vi "Fcurve_Create.vi"(0 "reference in":refnum<class "Fcurve.lvclass">, 1 "object name":string="Fcurve", 2 "Group metadata":T1, 5 "error in (no error)":errorcluster) -> (14 "reference out":refnum<class "Fcurve.lvclass">, 19 "error out":errorcluster)   [LabVIEW 2019, in "Fcurve.lvclass"]
doc: "Constructor."
uses:
  Fcurve.lvclass
  C:/Program Files (x86)/National Instruments/LabVIEW 2019/vi.lib/addons/_AddQ/G#Object/G#Object.lvclass
  TDMS_DataHandler_class/Fcurve Meta data.ctl
  <vilib>/addons/_AddQ/G#Object/utils/G#Object_CreateMethod.ctl
  <vilib>/addons/_AddQ/G#Object/G#Object.lvclass
  metadata_class/metadata.lvclass
  TDMS_DataHandler_class/TDMS_DataHandler.lvclass
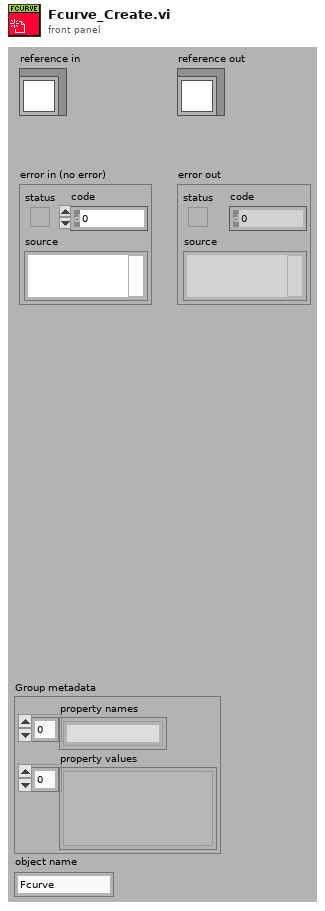
[diagram p1: front panel]
types:
  T1 = typedef "TDMS_DataHandler.lvclass/Fcurve Meta data.ctl" = cluster{"property names":string[], "property values":variant[]}
  T2 = typedef "G#Object.lvclass/G#Object_CreateMethod.ctl" = enum16{"Create", "Create or look up existing", "Look up existing"}
  T3 = typedef "Fcurve.lvclass/ObjectAttributesRef.ctl" = refnum<data-value>
  T4 = typedef "Fcurve.lvclass/ObjectAttributes.ctl" = cluster{"MyAttribute":dbl, "Fcurve Metadata":T5, "Contact Spread of dev":dbl, "Tau Delay (ms)":dbl, "Points of contact":dbl, "Def_wfm":cluster{"Max":dbl, "Min":dbl}, "Zpos_wfm":cluster{"Max":dbl, "Min":dbl}, "Contact stat?":bool, "Real AI dt (s)":dbl, "Decimation":cluster{"App":cluster{"Dec":i32, "apply":bool}, "Con":cluster{"Dec":i32, "apply":bool}, "Ret":cluster{"Dec":i32, "apply":bool}}, "Segment def[0]":dbl, "Segment Zpos[0]":dbl, "Raw Datum":waveform(dbl)[], "Group metadata":T1, "M_data obj":refnum<class "metadata.lvclass">, "Channel name(s)":string[], "Segment fcurve data":cluster{"X":dbl[], "Y":dbl[]}[], "Segment duration":cluster{"Start":i32, "Duration":i32}[], "Segment info":T6[], "Segment durations (S)":dbl[], "Segments Maxmin":T8[]}
  T5 = typedef "Fcurve.lvclass/Metadata.ctl" = cluster{"dt (us)":dbl, "Dec Factor":dbl, "Z piezo Sensitivity (nm/V)":dbl, "K (N/m)":dbl, "Sp (V)":dbl, "Contact (ms)":dbl, "Zpos contact":dbl, "Vel_app (nm/s)":dbl, "Vel_ret (nm/s)":dbl, "deltaV (nm)":dbl, "Def_V0 (v)":dbl, "Piezo gain":dbl, "invOLS (nm/V)":dbl}
  T6 = typedef "Fcurve.lvclass/Fcurve segments --cluster.ctl" = cluster{"type":T7, "nb points":i32, "dec factor":u32, "sampling rate (S/s)":u32}
  T7 = typedef "metadata.lvclass/Segment type--combobox.ctl" = string
  T8 = typedef "Fcurve.lvclass/Segment MaxMin --cluster.ctl" = cluster{"Def":cluster{"max value":dbl, "min value":dbl}, "Zpos":cluster{"max value":dbl, "min value":dbl}}
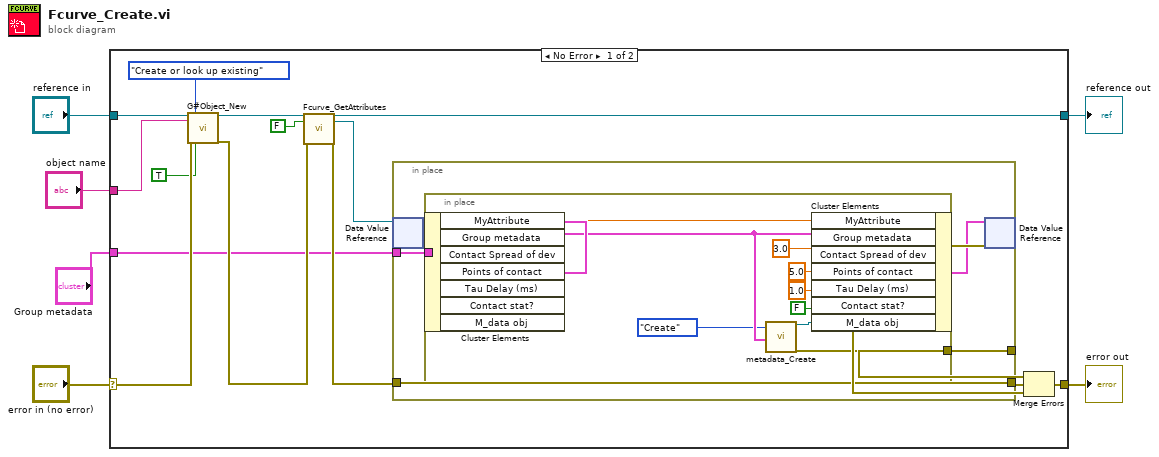
[diagram p0: block diagram]
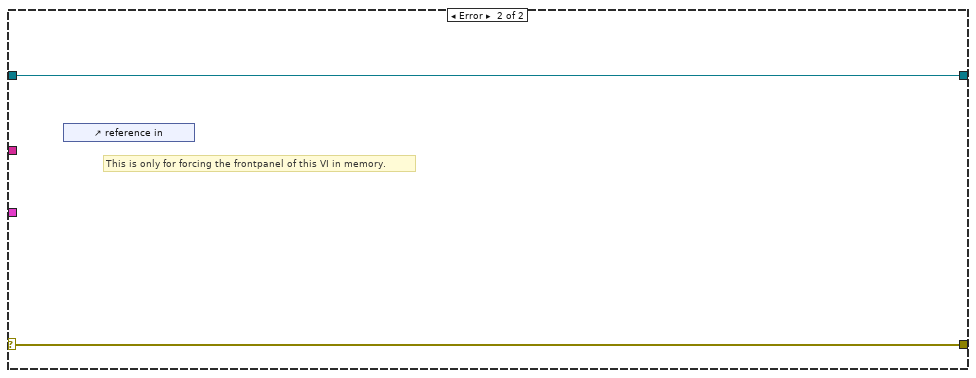
[diagram p2: hidden frame]
diagram:
  n1 = case shown="No Error" "error in (no error)" {
    selector: "error in (no error)" -> [w21 w38]
    tunnel: [w20 w38] -> w5
    tunnel: [w15 w37] -> w3
    tunnel: "reference in" -> [w22 w37]
    tunnel: "Group metadata" -> [w10 _]
    tunnel: "object name" -> [w9 _]
    frame No Error {
      n2 = call <vilib>:"G#Object_New.vi"("reference in"=w22, "object name"=w9, "error in (no error)"=w21, "create method"=G#Object_CreateMethod."Create or look up existing", "user counter (T)?"=TRUE ("User Counter")) -> ("reference out"=w16:refnum<class "Fcurve.lvclass">, "error out"=w14:errorcluster)  [unwired: 12 in, 1 out]
      n3 = call "Fcurve_GetAttributes.vi"("reference in"=w16, "return data? (T)"=FALSE ("return data"), "error in (no error)"=w14) -> ("reference out"=w15:refnum<class "Fcurve.lvclass">, "attributes ref"=w12:T3, "error out"=w13:errorcluster)  [unwired: 13 in, 1 out]
      n4 = in-place {
        in-place-border: w13 -> [w25]
        in-place-border: [w25] -> w18
        in-place-border: w10 -> [w24]
        in-place-border: [w23] -> w7
        n5 = in-place-dvr #1(w12) -> (w26:T4)  [unwired: 1 out]
        n6 = in-place {
          in-place-border: w24 -> [w30]
          in-place-border: [w29] -> w23
          n7 = in-place-cluster #2(w26) -> ("MyAttribute"=w36:dbl)  [unwired: 6 out]
          n8 = call "metadata_Create.vi"("Metadata"=w30, "create method"=G#Object_CreateMethod."Create") -> ("reference out"=w31:refnum<class "metadata.lvclass">, "error out"=w29:errorcluster)  [unwired: 16 in]
          n9 = in-place-cluster #2("MyAttribute"=w36, "Group metadata"=w30, "Contact Spread of dev"=3.0, "Points of contact"=5.0, "Tau Delay (ms)"=1.0, "Contact stat?"=FALSE, "M_data obj"=w31) -> (w27:T4)
        }
        n10 = in-place-dvr #1(w27) -> (w17:errorcluster)  [unwired: 1 out]
      }
      n11 = Merge Errors(w7, w18, w17) -> (w20:errorcluster)
    }
    frame Error {
      # "This is only for forcing the frontpanel of this VI in memory."
      n12 = control-ref of="reference in"() -> ()  [unwired: 1 out]
    }
  }
  "error out" <- w5
  "reference out" <- w3
